vi "binary to double array.vi"(8 "error in (no error)":errorcluster, 11 "Binary String":string) -> (0 "error out":errorcluster, 2 "Double Array":dbl[](array[numeric]), 3 "String":string)   [LabVIEW 2013]
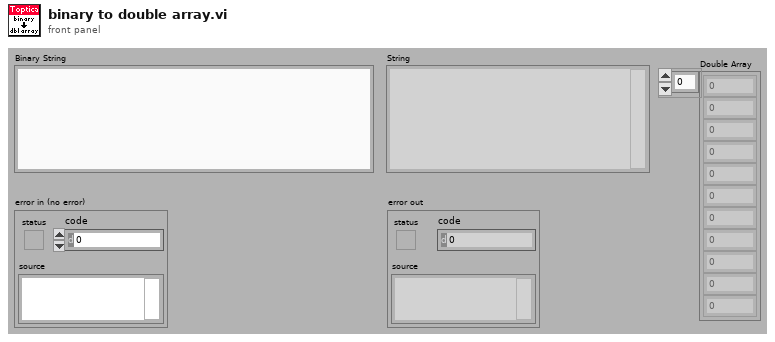
[diagram p1: front panel]
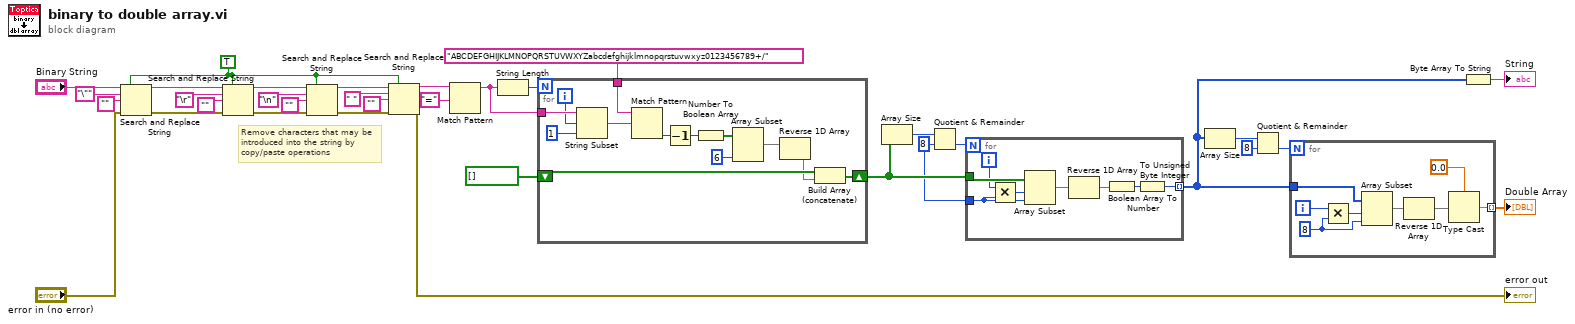
[diagram p0: block diagram]
diagram:
  w11 = TRUE ("replace all? (F)")
  w26 = 8 ("y")
  # "Remove characters that may be\nintroduced into the string by\ncopy/paste operations"
  n1 = Search and Replace String(replace all?=w11, input string="Binary String", search string="\"", replace string="", error in="error in (no error)") -> (result string=w13:string, error out=w1:errorcluster)  [unwired: 3 in, 2 out]
  n2 = Search and Replace String(replace all?=w11, input string=w13, search string="\r" ("replace string (\"\")"), replace string="", error in=w1) -> (result string=w21:string, error out=w19:errorcluster)  [unwired: 5 out]
  n3 = Search and Replace String(replace all?=w11, input string=w21, search string="\n" ("replace string (\"\")"), replace string="", error in=w19) -> (result string=w16:string, error out=w15:errorcluster)  [unwired: 5 out]
  n4 = Search and Replace String(replace all?=w11, input string=w16, search string=" " ("replace string (\"\")"), replace string="", error in=w15) -> (result string=w14:string, error out=→"error out":errorcluster)  [unwired: 5 out]
  n5 = Match Pattern(string=w14, regular expression="=") -> (before substring=w31:string)  [unwired: 4 out]
  n6 = String Length(string=w31) -> (length=w34:i32)
  n7 = for {
    N: w34 -> [_]
    tunnel: w31 -> [w47]
    tunnel: "ABCDEFGHIJKLMNOPQRSTUVWXYZabcdefghijklmnopqrstuvwxyz0123456789+/" -> [w44]
    shift-right: [w37] -> w27
    shift-left: bool[] [] -> [w36]
    i -> [w45]
    n8 = String Subset(string=w47, offset (0)=w45, length (rest)=1 ("length (rest)")) -> (substring=w43:string)
    n9 = Match Pattern(string=w44, regular expression=w43) -> (offset past match=w42:i32)  [unwired: 1 in, 3 out]
    n10 = Decrement(x=w42) -> (x-1=w41:i32)
    n11 = Number To Boolean Array(number=w41) -> (Boolean array=w40:bool[])
    n12 = Array Subset(array=w40, length=6) -> (w38:bool[])  [unwired: 1 in]
    n13 = Reverse 1D Array(array=w38) -> (reversed array=w35:bool[])
    n14 = Build Array (concatenate)(w36, w35) -> (w37:bool[])
  }
  n15 = Array Size(array=w27) -> (size(s)=w29:i32)
  n16 = Quotient & Remainder(x=w29, y=w26) -> (floor(x/y)=w28:i32)  [unwired: 1 out]
  n17 = for {
    N: w28 -> [_]
    tunnel: w27 -> [w55]
    tunnel: w26 -> [w54]
    tunnel: [w50] -> w5 mode=indexing
    i -> [w53]
    n18 = Multiply(x=w53, y=w54) -> (x*y=w48:i32)
    n19 = Array Subset(array=w55, index=w48, length=w54) -> (w52:bool[])
    n20 = Reverse 1D Array(array=w52) -> (reversed array=w49:bool[])
    n21 = Boolean Array To Number(Boolean array=w49) -> (number=w51:u32)
    n22 = To Unsigned Byte Integer(number=w51) -> (unsigned 8bit integer=w50:u8)
  }
  n23 = Array Size(array=w5) -> (size(s)=w7:i32)
  n24 = Quotient & Remainder(x=w7, y=8) -> (floor(x/y)=w6:i32)  [unwired: 1 out]
  n25 = for {
    N: w6 -> [_]
    tunnel: w5 -> [w59]
    tunnel: [w56] -> w8 mode=indexing
    i -> [w60]
    w61 = 8 ("length")
    n26 = Multiply(x=w60, y=w61) -> (x*y=w62:i32)
    n27 = Array Subset(array=w59, index=w62, length=w61) -> (w63:u8[])
    n28 = Reverse 1D Array(array=w63) -> (reversed array=w58:u8[])
    n29 = Type Cast(type=0.0, x=w58) -> (*(type *) &x=w56:dbl)
  }
  "Double Array" <- w8
  n30 = Byte Array To String(unsigned byte array=w5) -> (string=→"String":string)
